vi "Cypress.vi"() -> ()   [LabVIEW 2013]
uses:
  <vilib>/Rock Robotics/WPI/Joystick/WPI_JoystickAxis.ctl
  Robot Global Data.vi
  <vilib>/Rock Robotics/WPI/Joystick/WPI_JoystickGetSetRefNum.vi
panel:
  out "Driver Station Digital Input (1-8)[7]":bool
  out "Driver Station Digital Input (1-8)[6]":bool
  out "Driver Station Digital Input (1-8)[5]":bool
  out "Driver Station Digital Input (1-8)[4]":bool
  out "Driver Station Digital Input (1-8)[3]":bool
  out "Driver Station Digital Input (1-8)[2]":bool
  out "Driver Station Digital Input (1-8)[1]":bool
  out "Driver Station Digital Input (1-8)[0]":bool
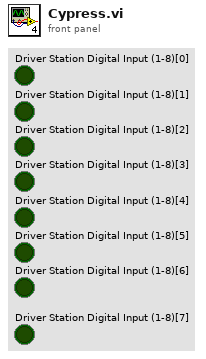
[diagram p1: front panel]
types:
  T1 = typedef "WPI_JoystickAxis.ctl" = enum16{"Axis 1", "Axis 2", "Axis 3", "Axis 4", "Axis 5", "Axis 6"}
  T2 = typedef "WPI_JoystickDevRef.ctl" = cluster{"Device":T3}
  T3 = typedef "WPI_JoystickDeviceEnum.ctl" = enum16{"USB 1", "USB 2", "USB 3", "USB 4", "Kinect 1", "Kinect 2"}
  T4 = typedef "WPI_JoystickButtonState.ctl" = cluster{"Button 1":bool, "Button 2":bool, "Button 3":bool, "Button 4":bool, "Button 5":bool, "Button 6":bool, "Button 7":bool, "Button 8":bool, "Button 9":bool, "Button 10":bool, "Button 11":bool, "Button 12":bool}
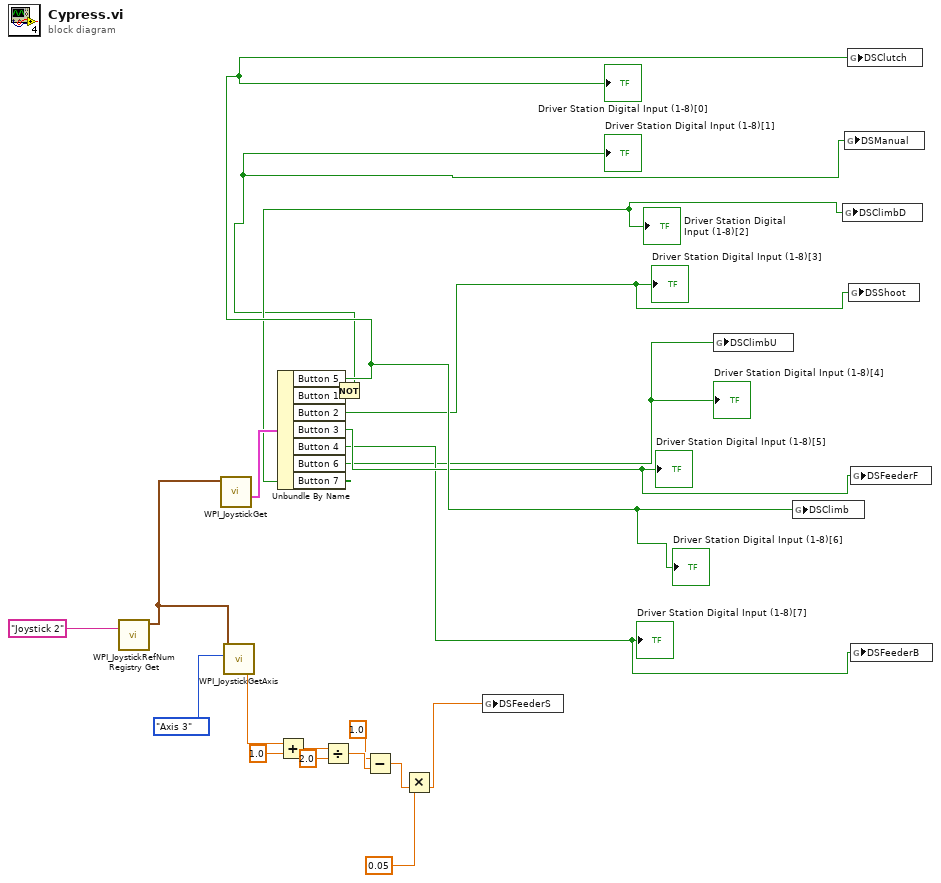
[diagram p0: block diagram]
diagram:
  n1 = call <vilib>:"WPI_JoystickRefNum Registry Get.vi"("refnum name"="Joystick 2") -> ("JoystickDevRef"=w19:T2)  [unwired: 9 in, 1 out]
  n2 = call <vilib>:"WPI_JoystickGet.vi"("JoystickDevRef"=w19) -> ("Buttons"=w16:T4)  [unwired: 4 in, 2 out]
  n3 = call <vilib>:"WPI_JoystickGetAxis.vi"("Axis"=WPI_JoystickAxis."Axis 3", "JoystickDevRef"=w19) -> ("Value"=w17:dbl)  [unwired: 8 in, 1 out]
  n4 = Unbundle By Name(w16) -> ("Button 5"=w14:bool, "Button 1"=w15:bool, "Button 2"=w13:bool, "Button 3"=w12:bool, "Button 4"=w11:bool, "Button 6"=w10:bool, "Button 7"=w9:bool)
  "Driver Station Digital Input (1-8)[0]" <- w14
  "Driver Station Digital Input (1-8)[2]" <- w9
  "Driver Station Digital Input (1-8)[3]" <- w13
  "Driver Station Digital Input (1-8)[4]" <- w10
  "Driver Station Digital Input (1-8)[5]" <- w12
  "Driver Station Digital Input (1-8)[6]" <- w14
  "Driver Station Digital Input (1-8)[7]" <- w11
  n5 = Add(x=w17, y=1.0) -> (x+y=w4:dbl)
  n6 = Divide(x=w4, y=2.0) -> (x/y=w2:dbl)
  n7 = Not(x=w15) -> (.not. x?=w8:bool)
  "Driver Station Digital Input (1-8)[1]" <- w8
  n8 = Subtract(x=1.0, y=w2) -> (x-y=w21:dbl)
  n9 = Multiply(x=0.05, y=w21) -> (x*y=w7:dbl)
  n10 = global write "Robot Global Data.vi" "DSFeederS"(w7) -> ()
  n11 = global write "Robot Global Data.vi" "DSClimbU"(w10) -> ()
  n12 = global write "Robot Global Data.vi" "DSClimb"(w14) -> ()
  n13 = global write "Robot Global Data.vi" "DSClimbD"(w9) -> ()
  n14 = global write "Robot Global Data.vi" "DSManual"(w8) -> ()
  n15 = global write "Robot Global Data.vi" "DSClutch"(w14) -> ()
  n16 = global write "Robot Global Data.vi" "DSShoot"(w13) -> ()
  n17 = global write "Robot Global Data.vi" "DSFeederF"(w12) -> ()
  n18 = global write "Robot Global Data.vi" "DSFeederB"(w11) -> ()
